vi "Threshold.vi"(8 "error in (no error)":errorcluster, 10 "Y Threshold":dbl, 11 "XY Graph":cluster{dbl[], dbl[]}(graph)={[0.0, 0.1, 0.2, 0.3, 0.4, 0.5, 0.6, 0.7, 0.8, 0.9, 1.0, 1.1, 1.2, 1.3, 1.4, 1.5, 1.6, 1.7, 1.8, 1.9, 2.0, 2.1, 2.2, 2.3, 2.4, 2.5, 2.6, 2.7, 2.8, 2.9, 3.0, 3.1, 3.2, 3.3, 3.4, 3.5, 3.6, 3.7, 3.8, 3.9, 4.0, 4.1, 4.2, 4.3, 4.4, 4.5, 4.6, 4.7, 4.8, 4.9, 5.0, 5.1, 5.2, 5.3, 5.4, 5.5, 5.6, 5.7, 5.8, 5.9, 6.0, 6.1, 6.2, 6.3, 6.4, 6.5, 6.6, 6.7, 6.8, 6.9, 7.0, 7.1, 7.2, 7.3, 7.4, 7.5, 7.6, 7.7, 7.8, 7.9, 8.0, 8.1, 8.2, 8.3, 8.4, 8.5, 8.6, 8.7, 8.8, 8.9, 9.0, 9.1, 9.2, 9.3, 9.4, 9.5, 9.6, 9.7, 9.8, 9.9], [0.0, 0.058505708301413106, 0.2829171087323842, 0.17580290044700042, 0.5652631586327654, 0.2939554510547109, 0.8464710238112635, 0.4135270521003817, 1.1259814171756577, 0.5350716224105259, 1.4032467423002988, 0.6591294927652218, 1.6777348647801915, 0.7862236845832966, 1.9489327770964686, 0.916856307818946, 2.216350131753071, 1.0515051028777236, 2.479522618351379, 1.1906201503682659, 2.7380151613447117, 1.3346207713498535, 2.991424916449261, 1.4838926394242713, 3.239384045074979, 1.638785124561257, 3.4815622476685313, 1.7996088869507916, 3.717669038521037, 1.9666337374537946, 3.9474557463736124, 2.1400867793863947, 4.1707172270424415, 2.3201508444355468, 4.387293276268293, 2.5069632334780243, 4.597069733060096, 2.700614770974847, 4.799979265933646, 2.9011491794536997, 4.996001836630619, 3.1085627783872916, 5.185164838124153, 3.3228045095415277, 5.367542905960566, 3.5437762886189335, 5.54325740423651, 3.7713336807755056, 5.712475589751728, 4.005286895358645, 5.875409460093868, 4.245402093015303, 6.032314293588873, 4.491402996168156, 6.183486891172347, 4.742972791768297, 6.329263532290352, 4.999756313219891, 6.470017658907569, 5.261362486449909, 6.606157303573275, 5.527367023276251, 6.738122279258352, 5.797315343525019, 6.866381150317158, 6.070725705771885, 6.991428005435734, 6.347092525145854, 7.113779054791005, 6.625889855345349, 7.233969074857203, 6.906575010885591, 7.352547725344128, 7.18859230463054, 7.470075763633021, 7.471376874868413, 7.587121182781622, 7.754358575573757, 7.704255299696349, 8.036965903062875, 7.822048820412799, 8.318629931999729, 7.9410679095833325, 8.59878823364433, 8.061870291241828, 8.876888749358798, 8.185001407699406, 9.15239359269276, 8.310990663026384, 9.42478275386421, 8.440347776990448, 9.693557681121064, 8.573559274563463, 9.9582447143198, 8.711085135172763, 10.218398347072213, 8.85335562477442, 10.473604294995038, 9.000768332566743, 10.723482348929684]}) -> (0 "error out":errorcluster, 2 "Indexes":dbl[](array[numeric]), 3 "X Values":dbl[](array[numeric]))   [LabVIEW 2019]
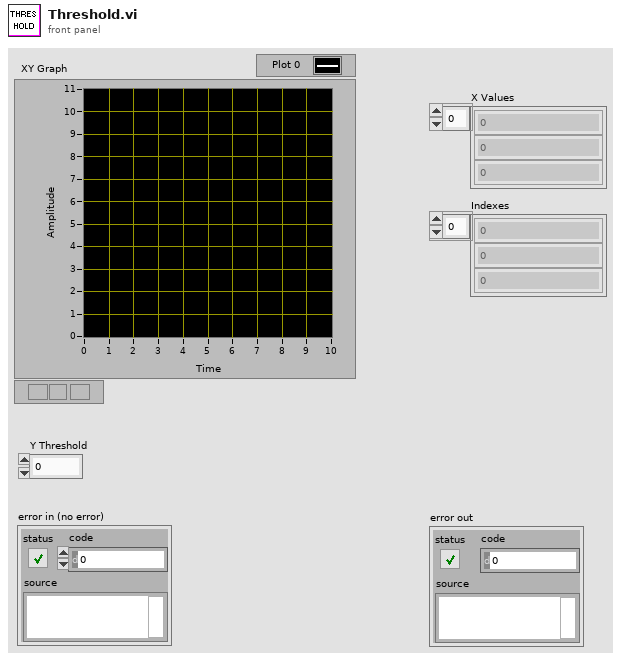
[diagram p1: front panel]
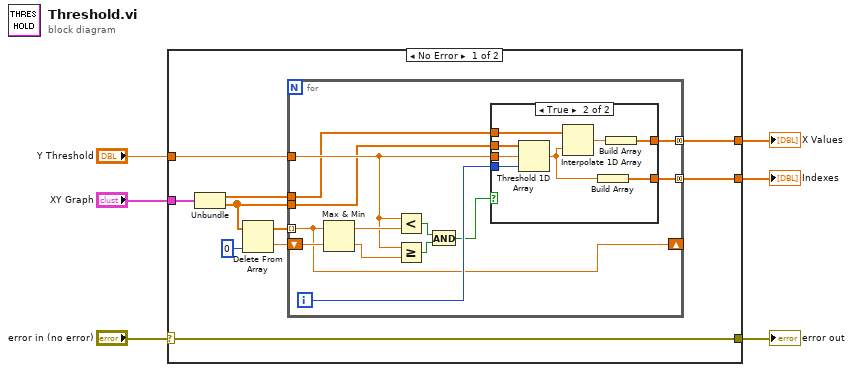
[diagram p0: block diagram]
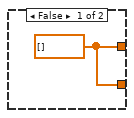
[diagram p2: hidden frame]
diagram:
  n1 = case shown="No Error" "error in (no error)" {
    selector: "error in (no error)" -> [w7 w39]
    tunnel: "XY Graph" -> [w11 _]
    tunnel: "Y Threshold" -> [w10 _]
    tunnel: [w9 _] -> w4
    tunnel: [w8 _] -> w3
    tunnel: [w7 w39] -> w2
    frame No Error {
      n2 = Unbundle(w11) -> (w16:dbl[], w12:dbl[])
      n3 = Delete From Array(array=w12, index=0) -> (deleted portion=w14:dbl, array with subset deleted=w13:dbl[])  [unwired: 1 in]
      n4 = for {
        tunnel: w16 -> [w21]
        tunnel: w13 -> [w20] mode=indexing
        shift-right: [w20] -> _
        shift-left: w14 -> [w25]
        tunnel: w10 -> [w24]
        tunnel: w12 -> [w23]
        tunnel: [w19] -> w9 mode=concatenating
        tunnel: [w17] -> w8 mode=concatenating
        i -> [w22]
        n5 = Max & Min(x=w20, y=w25) -> (max(x,y)=w27:dbl, min(x,y)=w26:dbl)
        n6 = Less?(x=w24, y=w27) -> (x < y?=w28:bool)
        n7 = Greater Or Equal?(x=w24, y=w26) -> (x >= y?=w29:bool)
        n8 = And(x=w28, y=w29) -> (x .and. y?=w18:bool)
        n9 = case shown="True" w18 {
          tunnel: w24 -> [_ w38]
          tunnel: w23 -> [_ w37]
          tunnel: w22 -> [_ w36]
          tunnel: w21 -> [_ w35]
          tunnel: [w30 w33] -> w19
          tunnel: [w30 w31] -> w17
          frame False {
            w30 = dbl[] []
          }
          frame True {
            n10 = Threshold 1D Array(1:w36, 2:w38, 3:w37) -> (0:w32:dbl)
            n11 = Interpolate 1D Array(1:w32, 2:w35) -> (0:w34:dbl)
            n12 = Build Array(w32) -> (w31:dbl[])
            n13 = Build Array(w34) -> (w33:dbl[])
          }
        }
      }
    }
    frame Error {
    }
  }
  "X Values" <- w4
  "Indexes" <- w3
  "error out" <- w2
